vi "Variant_to_Path.vi"(8 "Error in":errorcluster, 11 "Value (in)":variant) -> (0 "Error out":errorcluster, 2 "Value (string)":string, 3 "Value (out)":path)   [LabVIEW 2012]
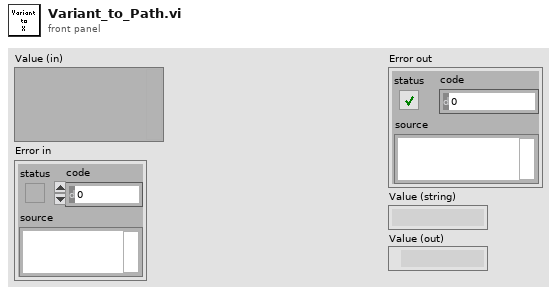
[diagram p1: front panel]
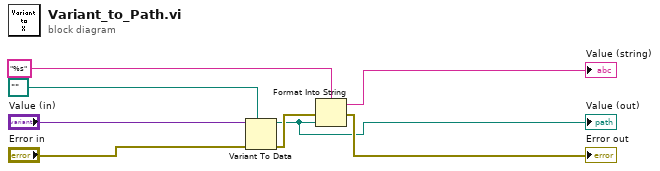
[diagram p0: block diagram]
diagram:
  n1 = Variant To Data(error in="Error in", type=path "" ("path"), Variant="Value (in)") -> (data=w1:path, error out=w8:errorcluster)
  "Value (out)" <- w1
  n2 = Format Into String(format string="%s", error in=w8, w1) -> (resulting string=→"Value (string)":string, error out=→"Error out":errorcluster)  [unwired: 1 in]
